vi "SaveControlValues.vi"(0 "XML File Path":path, 3 "error in (no error)":errorcluster) -> (10 "error out":errorcluster)   [LabVIEW 2024]
doc: "Use this as a SubVI inside a VI that you want to save and load the controls/indicators from. Refer to the <B>SaveLoadControlValuesDemo.vi</B> to see a demonstration of how to use this VI.\n\n<B>Dat file</B> specifies the name and path of the *.dat file. If the control is empty, the default file will be used (see block diagram for further information).\n\nIf names are specified in <B>Specific controls/indicators</B>, the <B>Controls or indicators?</B> will be ignored."
uses:
  <vilib>/NI/GXML/GXML.lvlib
panel:
  out "Concatenated GXML String":string
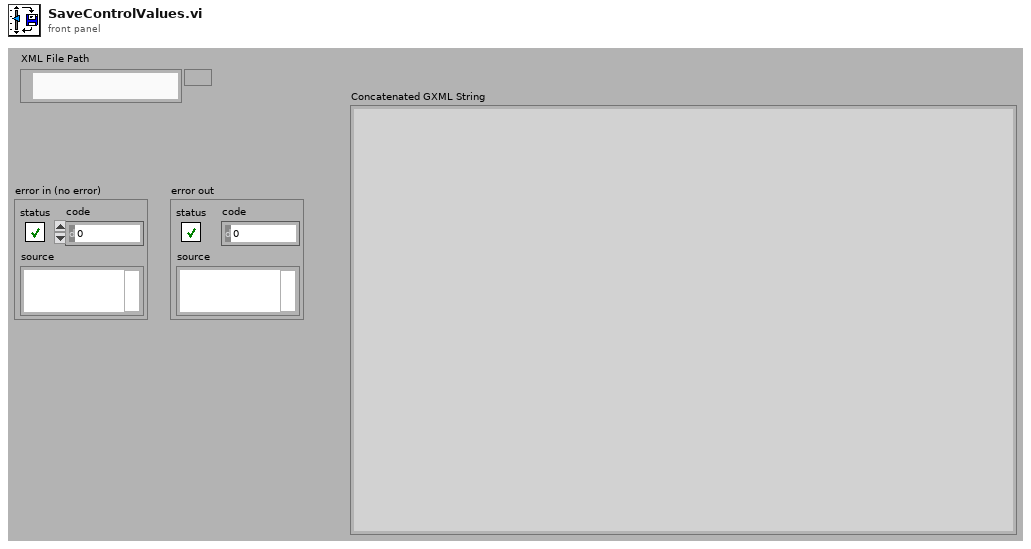
[diagram p1: front panel]
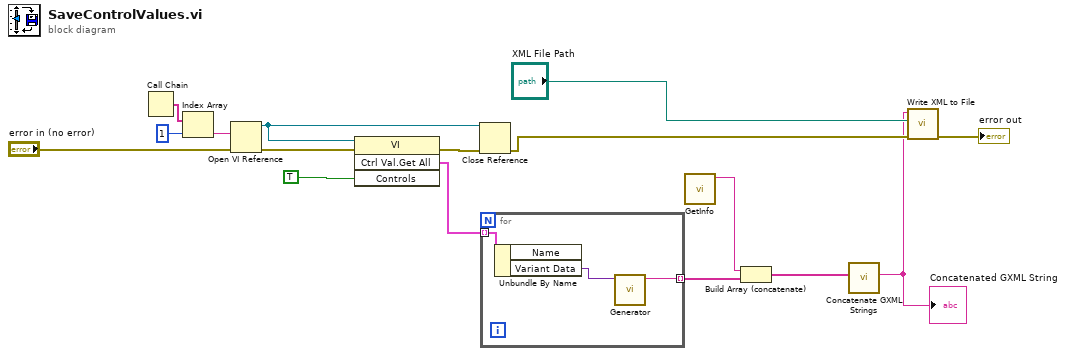
[diagram p0: block diagram]
diagram:
  n1 = Call Chain() -> (call chain=w15:string[])
  n2 = Index Array(array=w15, index=1) -> (element=w11:string)
  n3 = Open VI Reference(vi path=w11, error in (no error)="error in (no error)") -> (vi reference=w12:refnum<vi>, error out=w13:errorcluster)  [unwired: 4 in]
  n4 = invoke class="VI" method="Ctrl Val.Get All"(reference=w12, error in=w13, "Controls"=TRUE) -> (error out=w9:errorcluster, "Get All Control Values Variant"=w8:cluster{"Name":string, "Variant Data":variant}[])  [unwired: 1 in, 2 out]
  n5 = Close Reference(reference=w12, error in (no error)=w9) -> (error out=w7:errorcluster)
  n6 = for {
    tunnel: w8 -> [w19] mode=indexing
    tunnel: [w17] -> w2 mode=indexing
    n7 = Unbundle By Name(w19) -> ("Variant Data"=w18:variant)  [unwired: 1 out]
    n8 = call <vilib>:"Generator.vi"("Variant"=w18) -> ("XML String Out"=w17:string)  [unwired: 9 in, 1 out]
  }
  n9 = call "GetInfo.vi"() -> ("concatenated string"=w1:string)  [unwired: 11 in]
  n10 = Build Array (concatenate)(w1, w2) -> (w3:string[])
  n11 = call <vilib>:"Concatenate GXML Strings.vi"("GXML Strings"=w3) -> ("Concatenated GXML String"=w4:string)  [unwired: 9 in, 1 out]
  "Concatenated GXML String" <- w4
  n12 = call <vilib>:"Write XML to File.vi"("error in"=w7, "XML File Path"="XML File Path", "XML Input"=w4) -> ("error out"=→"error out":errorcluster)  [unwired: 8 in]
